vi "Send Bark Message.vi"(8 "Message":string, 9 "Title":string, 10 "Group":string, 11 "Url":string) -> ()   [LabVIEW 2016, in "Bark.lvlib" / "Bark.lvclass"]
uses:
  Bark.lvclass
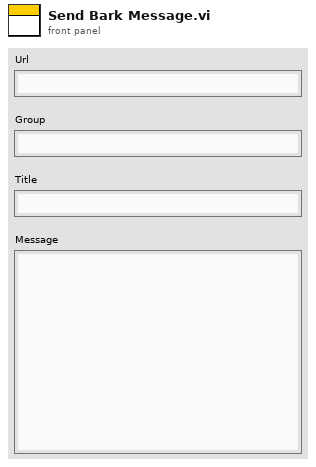
[diagram p1: front panel]
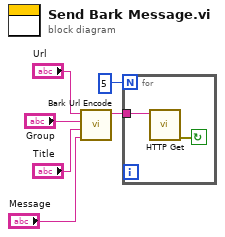
[diagram p0: block diagram]
diagram:
  n1 = call "Bark Url Encode.vi"("Message"="Message", "Title"="Title", "Group"="Group", "Url"="Url") -> ("UrlEncode"=w6:string)  [unwired: 7 in]
  n2 = for {
    N: 5 -> [_]
    tunnel: w6 -> [w8]
    stop <- w7 continue-if-true
    n3 = call "HTTP Get.vi"("url"=w8) -> ("error out"=w7:errorcluster)  [unwired: 10 in]
  }
